vi "zmq_poll.vi"   [LabVIEW 2015, in "zeromq.lvlib" / "zmq_socket.lvclass"]
uses:
  zmq_socket.lvclass
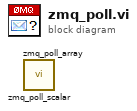
[diagram p0: block diagram]
diagram:
  n1 = call "zmq_poll_scalar.vi"() -> ()  [unwired: 4 in, 4 out]
  n2 = call "zmq_poll_array.vi"() -> ()  [unwired: 4 in, 4 out]
